vi "WILT Step Drying Clothes 3.vi"(6 "Delay After Cutout (sec)":dbl=5.0 format="%#_13g", 7 "Station Number in":u32, 8 "Error In":errorcluster, 9 "Current Threshold":dbl=1.0 format="%#_13g", 10 "Station Test State Cluster":T1, 11 "Dryer Input":T3 {"Night Cycle Count" format="%04d"; "Day Cycle Count" format="%04d"}) -> (0 "Error Out":errorcluster, 2 "Step 2 Output":T1, 3 "Dryer Output":T3 {"Night Cycle Count" format="%04d"; "Day Cycle Count" format="%04d"})   [LabVIEW 2016]
uses:
  Type Definitions/WILT Dryer.ctl
  Type Definitions/WILT Dryer Details.ctl
  Type Definitions/WILT Agilent Channel Definition.ctl
  Type Definitions/WILT DAQ Data.ctl
  Type Definitions/WILT Station Test State Cluster.ctl
  Type Definitions/WILT Dryer Test State.ctl
  Globals/WILT Globals Main Program.vi
panel:
  # "Day"
  # "Night"
  # "Day"
  # "Night"
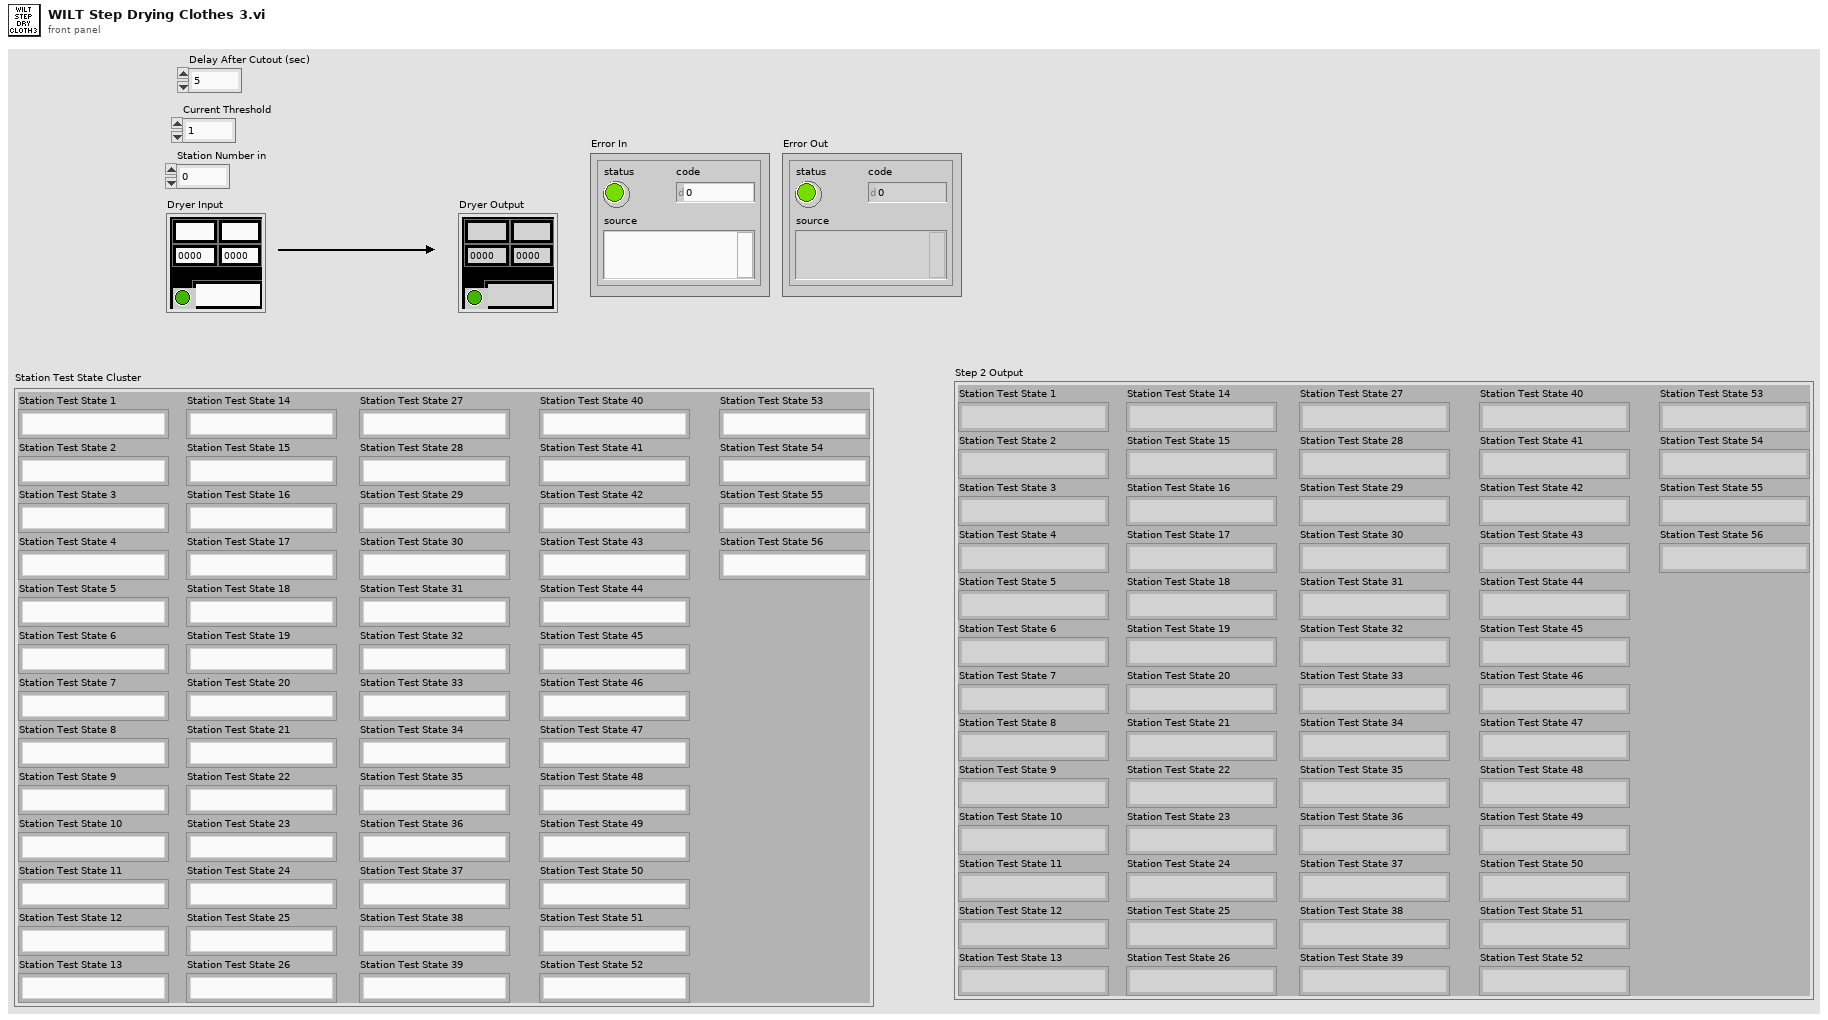
[diagram p1: front panel]
types:
  T1 = typedef "WILT Station Test State Cluster.ctl" = cluster{"Station Test State 1":T2, "Station Test State 2":T2, "Station Test State 3":T2, "Station Test State 4":T2, "Station Test State 5":T2, "Station Test State 6":T2, "Station Test State 7":T2, "Station Test State 8":T2, "Station Test State 9":T2, "Station Test State 10":T2, "Station Test State 11":T2, "Station Test State 12":T2, "Station Test State 13":T2, "Station Test State 14":T2, "Station Test State 15":T2, "Station Test State 16":T2, "Station Test State 17":T2, "Station Test State 18":T2, "Station Test State 19":T2, "Station Test State 20":T2, "Station Test State 21":T2, "Station Test State 22":T2, "Station Test State 23":T2, "Station Test State 24":T2, "Station Test State 25":T2, "Station Test State 26":T2, "Station Test State 27":T2, "Station Test State 28":T2, "Station Test State 29":T2, "Station Test State 30":T2, "Station Test State 31":T2, "Station Test State 32":T2, "Station Test State 33":T2, "Station Test State 34":T2, "Station Test State 35":T2, "Station Test State 36":T2, "Station Test State 37":T2, "Station Test State 38":T2, "Station Test State 39":T2, "Station Test State 40":T2, "Station Test State 41":T2, "Station Test State 42":T2, "Station Test State 43":T2, "Station Test State 44":T2, "Station Test State 45":T2, "Station Test State 46":T2, "Station Test State 47":T2, "Station Test State 48":T2, "Station Test State 49":T2, "Station Test State 50":T2, "Station Test State 51":T2, "Station Test State 52":T2, "Station Test State 53":T2, "Station Test State 54":T2, "Station Test State 55":T2, "Station Test State 56":T2}
  T2 = typedef "WILT Dryer Test State.ctl" = enum16{"No Serial Number", "Waiting for Dryer To Start", "Drying Clothes", "Water Injection 1 (On)", "Water Injection 1 Timer", "Water Injection 1 (Off)", "Pause Dryer", "Sending Start Stop CMD", "Pause Dryer 2", "Sending Start Stop CMD 2", "Drying Clothes 2", "Water Injection 2 (On)", "Water Injection 2 Timer", "Water Injection 2 (Off)", "Drying Clothes 3", "Cooling Down", "Sending Start Stop CMD 3", "Increment Cycle"}
  T3 = typedef "WILT Dryer.ctl" = cluster{"Lab ID":string, "Day Cycle Count":i32, "Station Label":string, "Dryer Details":T4, "Status Color":u32, "Invisible Button":bool, "Night Cycle Count":i32, "Station Index":i32, "Cycle Index":string, "Audit Alert":bool, "Agilent Channel Definition":T5, "DAQ Data":T6}
  T4 = typedef "WILT Dryer Details.ctl" = cluster{"Station":string, "Lab ID":string, "TR Number":string}
  T5 = typedef "WILT Agilent Channel Definition.ctl" = cluster{"Channel":string, "Station":string, "Label":string, "Agilent Station":string, "Data":dbl}
  T6 = typedef "WILT DAQ Data.ctl" = cluster{"L1 Current":dbl, "L2 Current":dbl, "Temperature  Deg F (TC)":dbl, "Volts":dbl, "Volts (208)":dbl, "SW (208)":dbl}
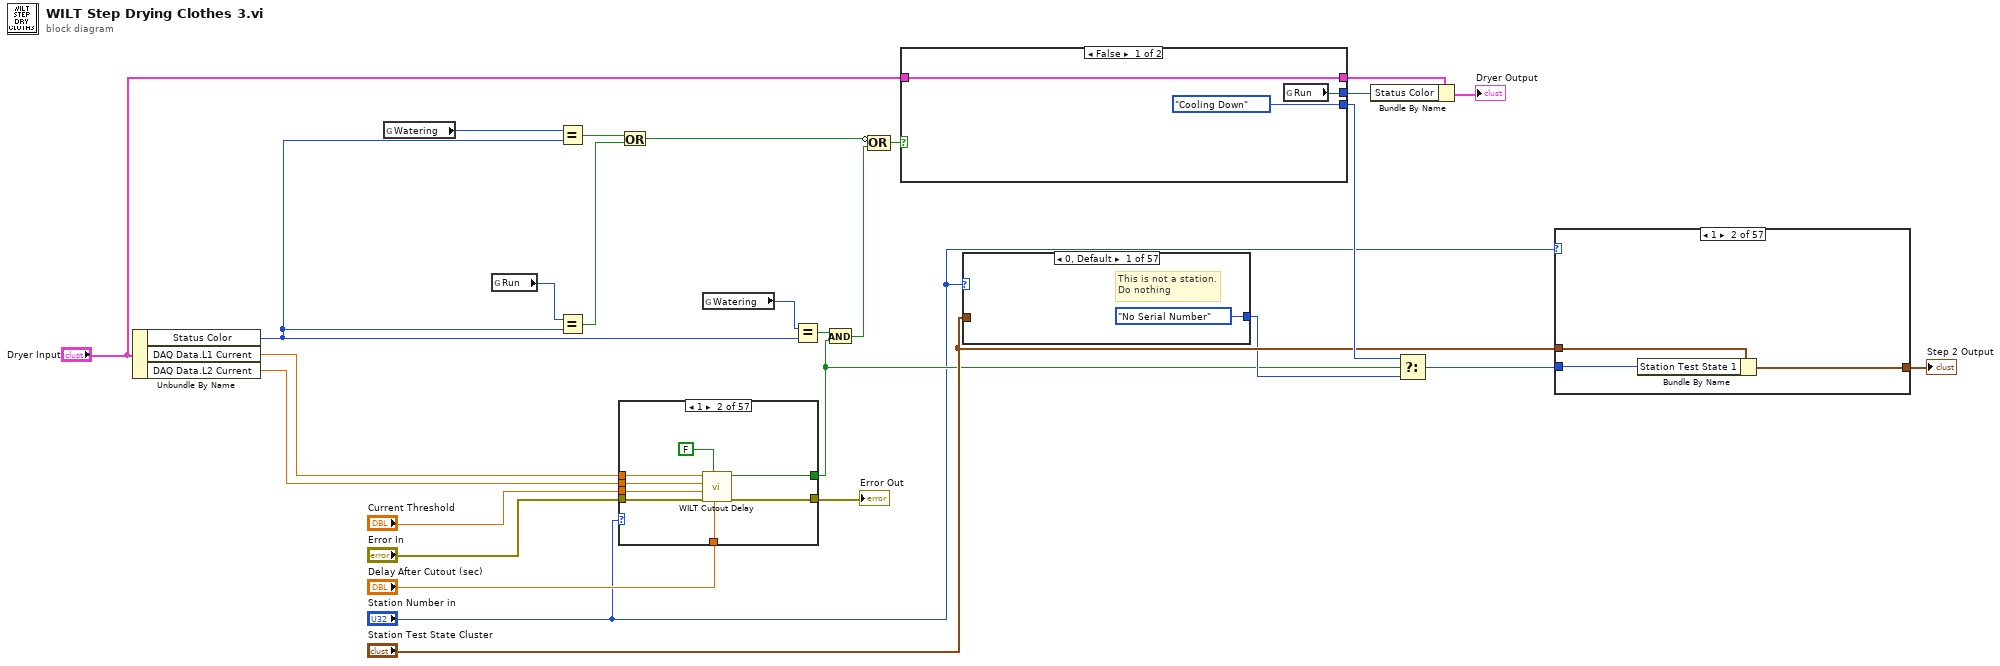
[diagram p0: block diagram]
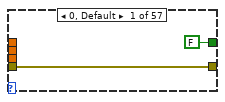
[diagram p2: hidden frame]
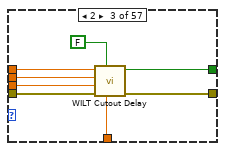
[diagram p3: hidden frame]
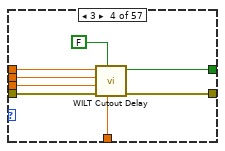
[diagram p4: hidden frame]
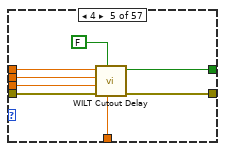
[diagram p5: hidden frame]
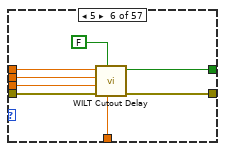
[diagram p6: hidden frame]
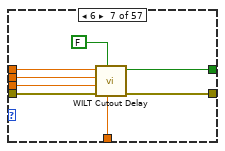
[diagram p7: hidden frame]
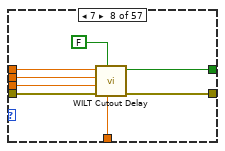
[diagram p8: hidden frame]
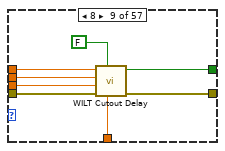
[diagram p9: hidden frame]
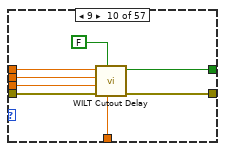
[diagram p10: hidden frame]
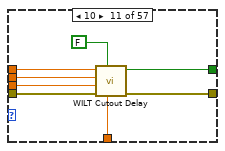
[diagram p11: hidden frame]
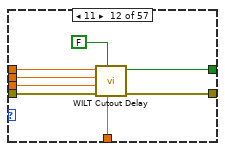
[diagram p12: hidden frame]
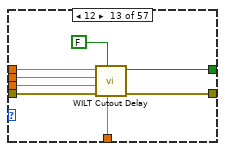
[diagram p13: hidden frame]
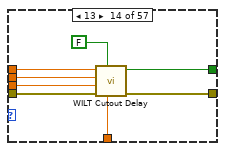
[diagram p14: hidden frame]
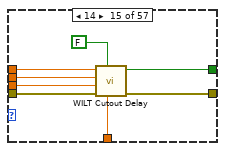
[diagram p15: hidden frame]
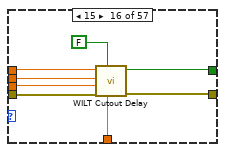
[diagram p16: hidden frame]
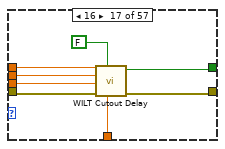
[diagram p17: hidden frame]
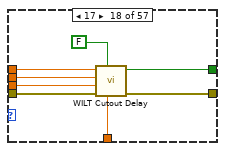
[diagram p18: hidden frame]
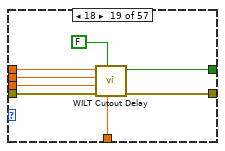
[diagram p19: hidden frame]
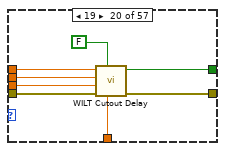
[diagram p20: hidden frame]
diagram:
  n1 = Unbundle By Name("Dryer Input") -> ("Status Color"=w11:u32, "DAQ Data.L1 Current"=w25:dbl, "DAQ Data.L2 Current"=w24:dbl)
  n2 = global read "WILT Globals Main Program.vi" "Watering"() -> (w13:u32)
  n3 = global read "WILT Globals Main Program.vi" "Run"() -> (w12:u32)
  n4 = Equal?(x=w13, y=w11) -> (x = y?=w10:bool)
  n5 = Equal?(x=w12, y=w11) -> (x = y?=w9:bool)
  n6 = case shown="1" "Station Number in" {
    tunnel: "Current Threshold" -> [_ w37 w40 w48 w59 w67 w75 w83 w91 w99 w107 w115 w123 w131 w139 w144 w155 w163 w171 w179 w187 w195 w203 w211 w219 w227 w235 w243 w251 w259 w267 w275 w283 w291 w299 w307 w315 w323 w331 w339 w347 w355 w363 w371 w379 w387 w395 w403 w411 w419 w427 w435 w443 w451 w459 w467 w475]
    tunnel: w25 -> [_ w36 w42 w50 w61 w69 w77 w85 w93 w101 w109 w117 w125 w133 w141 w146 w157 w165 w173 w181 w189 w197 w205 w213 w221 w229 w237 w245 w253 w261 w269 w277 w285 w293 w301 w309 w317 w325 w333 w341 w349 w357 w365 w373 w381 w389 w397 w405 w413 w421 w429 w437 w445 w453 w461 w469 w477]
    tunnel: w24 -> [_ w35 w41 w49 w60 w68 w76 w84 w92 w100 w108 w116 w124 w132 w140 w145 w156 w164 w172 w180 w188 w196 w204 w212 w220 w228 w236 w244 w252 w260 w268 w276 w284 w292 w300 w308 w316 w324 w332 w340 w348 w356 w364 w372 w380 w388 w396 w404 w412 w420 w428 w436 w444 w452 w460 w468 w476]
    tunnel: [FALSE ("Delayed Trigger") w34 w39 w51 w55 w64 w72 w79 w88 w96 w104 w111 w121 w129 w137 w147 w152 w160 w168 w177 w184 w191 w200 w207 w216 w224 w231 w240 w248 w256 w264 w271 w279 w287 w295 w303 w312 w319 w327 w336 w343 w351 w359 w367 w376 w384 w391 w400 w407 w416 w424 w432 w440 w448 w456 w464 w471] -> w16
    tunnel: "Error In" -> [w29 w33 w45 w53 w58 w66 w74 w82 w90 w98 w106 w114 w122 w130 w138 w149 w154 w162 w170 w178 w186 w194 w202 w210 w218 w226 w234 w242 w250 w258 w266 w274 w282 w290 w298 w306 w314 w322 w330 w338 w346 w354 w362 w370 w378 w386 w394 w402 w410 w418 w426 w434 w442 w450 w458 w466 w474]
    tunnel: [w29 w32 w44 w52 w56 w65 w71 w80 w89 w97 w103 w112 w120 w128 w136 w148 w153 w161 w169 w176 w185 w192 w199 w208 w217 w223 w232 w241 w249 w257 w265 w272 w280 w288 w296 w304 w313 w320 w328 w337 w344 w352 w360 w368 w377 w385 w392 w401 w408 w417 w425 w433 w441 w449 w457 w465 w472] -> w3
    tunnel: "Delay After Cutout (sec)" -> [_ w31 w43 w47 w57 w63 w73 w81 w87 w95 w105 w113 w119 w127 w135 w143 w151 w159 w167 w175 w183 w193 w201 w209 w215 w225 w233 w239 w247 w255 w263 w273 w281 w289 w297 w305 w311 w321 w329 w335 w345 w353 w361 w369 w375 w383 w393 w399 w409 w415 w423 w431 w439 w447 w455 w463 w473]
    frame 0, Default {
    }
    frame 1 {
      n7 = call "WILT Cutout Delay.vi"("Delay After Cutout (sec)"=w31, "Cut-In?"=FALSE, "Error In"=w33, "Current Threshold"=w37, "L2 Current"=w35, "L1 Current"=w36) -> ("Error Out"=w32:errorcluster, "Delayed Trigger"=w34:bool)  [unwired: 2 in, 2 out]
    }
    frame 2 {
      n8 = call "WILT Cutout Delay.vi"("Delay After Cutout (sec)"=w43, "Cut-In?"=FALSE, "Error In"=w45, "Current Threshold"=w40, "L2 Current"=w41, "L1 Current"=w42) -> ("Error Out"=w44:errorcluster, "Delayed Trigger"=w39:bool)  [unwired: 2 in, 2 out]
    }
    frame 3 {
      n9 = call "WILT Cutout Delay.vi"("Delay After Cutout (sec)"=w47, "Cut-In?"=FALSE, "Error In"=w53, "Current Threshold"=w48, "L2 Current"=w49, "L1 Current"=w50) -> ("Error Out"=w52:errorcluster, "Delayed Trigger"=w51:bool)  [unwired: 2 in, 2 out]
    }
    frame 4 {
      n10 = call "WILT Cutout Delay.vi"("Delay After Cutout (sec)"=w57, "Cut-In?"=FALSE, "Error In"=w58, "Current Threshold"=w59, "L2 Current"=w60, "L1 Current"=w61) -> ("Error Out"=w56:errorcluster, "Delayed Trigger"=w55:bool)  [unwired: 2 in, 2 out]
    }
    frame 5 {
      n11 = call "WILT Cutout Delay.vi"("Delay After Cutout (sec)"=w63, "Cut-In?"=FALSE, "Error In"=w66, "Current Threshold"=w67, "L2 Current"=w68, "L1 Current"=w69) -> ("Error Out"=w65:errorcluster, "Delayed Trigger"=w64:bool)  [unwired: 2 in, 2 out]
    }
    frame 6 {
      n12 = call "WILT Cutout Delay.vi"("Delay After Cutout (sec)"=w73, "Cut-In?"=FALSE, "Error In"=w74, "Current Threshold"=w75, "L2 Current"=w76, "L1 Current"=w77) -> ("Error Out"=w71:errorcluster, "Delayed Trigger"=w72:bool)  [unwired: 2 in, 2 out]
    }
    frame 7 {
      n13 = call "WILT Cutout Delay.vi"("Delay After Cutout (sec)"=w81, "Cut-In?"=FALSE, "Error In"=w82, "Current Threshold"=w83, "L2 Current"=w84, "L1 Current"=w85) -> ("Error Out"=w80:errorcluster, "Delayed Trigger"=w79:bool)  [unwired: 2 in, 2 out]
    }
    frame 8 {
      n14 = call "WILT Cutout Delay.vi"("Delay After Cutout (sec)"=w87, "Cut-In?"=FALSE, "Error In"=w90, "Current Threshold"=w91, "L2 Current"=w92, "L1 Current"=w93) -> ("Error Out"=w89:errorcluster, "Delayed Trigger"=w88:bool)  [unwired: 2 in, 2 out]
    }
    frame 9 {
      n15 = call "WILT Cutout Delay.vi"("Delay After Cutout (sec)"=w95, "Cut-In?"=FALSE, "Error In"=w98, "Current Threshold"=w99, "L2 Current"=w100, "L1 Current"=w101) -> ("Error Out"=w97:errorcluster, "Delayed Trigger"=w96:bool)  [unwired: 2 in, 2 out]
    }
    frame 10 {
      n16 = call "WILT Cutout Delay.vi"("Delay After Cutout (sec)"=w105, "Cut-In?"=FALSE, "Error In"=w106, "Current Threshold"=w107, "L2 Current"=w108, "L1 Current"=w109) -> ("Error Out"=w103:errorcluster, "Delayed Trigger"=w104:bool)  [unwired: 2 in, 2 out]
    }
    frame 11 {
      n17 = call "WILT Cutout Delay.vi"("Delay After Cutout (sec)"=w113, "Cut-In?"=FALSE, "Error In"=w114, "Current Threshold"=w115, "L2 Current"=w116, "L1 Current"=w117) -> ("Error Out"=w112:errorcluster, "Delayed Trigger"=w111:bool)  [unwired: 2 in, 2 out]
    }
    frame 12 {
      n18 = call "WILT Cutout Delay.vi"("Delay After Cutout (sec)"=w119, "Cut-In?"=FALSE, "Error In"=w122, "Current Threshold"=w123, "L2 Current"=w124, "L1 Current"=w125) -> ("Error Out"=w120:errorcluster, "Delayed Trigger"=w121:bool)  [unwired: 2 in, 2 out]
    }
    frame 13 {
      n19 = call "WILT Cutout Delay.vi"("Delay After Cutout (sec)"=w127, "Cut-In?"=FALSE, "Error In"=w130, "Current Threshold"=w131, "L2 Current"=w132, "L1 Current"=w133) -> ("Error Out"=w128:errorcluster, "Delayed Trigger"=w129:bool)  [unwired: 2 in, 2 out]
    }
    frame 14 {
      n20 = call "WILT Cutout Delay.vi"("Delay After Cutout (sec)"=w135, "Cut-In?"=FALSE, "Error In"=w138, "Current Threshold"=w139, "L2 Current"=w140, "L1 Current"=w141) -> ("Error Out"=w136:errorcluster, "Delayed Trigger"=w137:bool)  [unwired: 2 in, 2 out]
    }
    frame 15 {
      n21 = call "WILT Cutout Delay.vi"("Delay After Cutout (sec)"=w143, "Cut-In?"=FALSE, "Error In"=w149, "Current Threshold"=w144, "L2 Current"=w145, "L1 Current"=w146) -> ("Error Out"=w148:errorcluster, "Delayed Trigger"=w147:bool)  [unwired: 2 in, 2 out]
    }
    frame 16 {
      n22 = call "WILT Cutout Delay.vi"("Delay After Cutout (sec)"=w151, "Cut-In?"=FALSE, "Error In"=w154, "Current Threshold"=w155, "L2 Current"=w156, "L1 Current"=w157) -> ("Error Out"=w153:errorcluster, "Delayed Trigger"=w152:bool)  [unwired: 2 in, 2 out]
    }
    frame 17 {
      n23 = call "WILT Cutout Delay.vi"("Delay After Cutout (sec)"=w159, "Cut-In?"=FALSE, "Error In"=w162, "Current Threshold"=w163, "L2 Current"=w164, "L1 Current"=w165) -> ("Error Out"=w161:errorcluster, "Delayed Trigger"=w160:bool)  [unwired: 2 in, 2 out]
    }
    frame 18 {
      n24 = call "WILT Cutout Delay.vi"("Delay After Cutout (sec)"=w167, "Cut-In?"=FALSE, "Error In"=w170, "Current Threshold"=w171, "L2 Current"=w172, "L1 Current"=w173) -> ("Error Out"=w169:errorcluster, "Delayed Trigger"=w168:bool)  [unwired: 2 in, 2 out]
    }
    frame 19 {
      n25 = call "WILT Cutout Delay.vi"("Delay After Cutout (sec)"=w175, "Cut-In?"=FALSE, "Error In"=w178, "Current Threshold"=w179, "L2 Current"=w180, "L1 Current"=w181) -> ("Error Out"=w176:errorcluster, "Delayed Trigger"=w177:bool)  [unwired: 2 in, 2 out]
    }
    frame 20 {
      n26 = call "WILT Cutout Delay.vi"("Delay After Cutout (sec)"=w183, "Cut-In?"=FALSE, "Error In"=w186, "Current Threshold"=w187, "L2 Current"=w188, "L1 Current"=w189) -> ("Error Out"=w185:errorcluster, "Delayed Trigger"=w184:bool)  [unwired: 2 in, 2 out]
    }
    frame 21 {
      n27 = call "WILT Cutout Delay.vi"("Delay After Cutout (sec)"=w193, "Cut-In?"=FALSE, "Error In"=w194, "Current Threshold"=w195, "L2 Current"=w196, "L1 Current"=w197) -> ("Error Out"=w192:errorcluster, "Delayed Trigger"=w191:bool)  [unwired: 2 in, 2 out]
    }
    frame 22 {
      n28 = call "WILT Cutout Delay.vi"("Delay After Cutout (sec)"=w201, "Cut-In?"=FALSE, "Error In"=w202, "Current Threshold"=w203, "L2 Current"=w204, "L1 Current"=w205) -> ("Error Out"=w199:errorcluster, "Delayed Trigger"=w200:bool)  [unwired: 2 in, 2 out]
    }
    frame 23 {
      n29 = call "WILT Cutout Delay.vi"("Delay After Cutout (sec)"=w209, "Cut-In?"=FALSE, "Error In"=w210, "Current Threshold"=w211, "L2 Current"=w212, "L1 Current"=w213) -> ("Error Out"=w208:errorcluster, "Delayed Trigger"=w207:bool)  [unwired: 2 in, 2 out]
    }
    frame 24 {
      n30 = call "WILT Cutout Delay.vi"("Delay After Cutout (sec)"=w215, "Cut-In?"=FALSE, "Error In"=w218, "Current Threshold"=w219, "L2 Current"=w220, "L1 Current"=w221) -> ("Error Out"=w217:errorcluster, "Delayed Trigger"=w216:bool)  [unwired: 2 in, 2 out]
    }
    frame 25 {
      n31 = call "WILT Cutout Delay.vi"("Delay After Cutout (sec)"=w225, "Cut-In?"=FALSE, "Error In"=w226, "Current Threshold"=w227, "L2 Current"=w228, "L1 Current"=w229) -> ("Error Out"=w223:errorcluster, "Delayed Trigger"=w224:bool)  [unwired: 2 in, 2 out]
    }
    frame 26 {
      n32 = call "WILT Cutout Delay.vi"("Delay After Cutout (sec)"=w233, "Cut-In?"=FALSE, "Error In"=w234, "Current Threshold"=w235, "L2 Current"=w236, "L1 Current"=w237) -> ("Error Out"=w232:errorcluster, "Delayed Trigger"=w231:bool)  [unwired: 2 in, 2 out]
    }
    frame 27 {
      n33 = call "WILT Cutout Delay.vi"("Delay After Cutout (sec)"=w239, "Cut-In?"=FALSE, "Error In"=w242, "Current Threshold"=w243, "L2 Current"=w244, "L1 Current"=w245) -> ("Error Out"=w241:errorcluster, "Delayed Trigger"=w240:bool)  [unwired: 2 in, 2 out]
    }
    frame 28 {
      n34 = call "WILT Cutout Delay.vi"("Delay After Cutout (sec)"=w247, "Cut-In?"=FALSE, "Error In"=w250, "Current Threshold"=w251, "L2 Current"=w252, "L1 Current"=w253) -> ("Error Out"=w249:errorcluster, "Delayed Trigger"=w248:bool)  [unwired: 2 in, 2 out]
    }
    frame 29 {
      n35 = call "WILT Cutout Delay.vi"("Delay After Cutout (sec)"=w255, "Cut-In?"=FALSE, "Error In"=w258, "Current Threshold"=w259, "L2 Current"=w260, "L1 Current"=w261) -> ("Error Out"=w257:errorcluster, "Delayed Trigger"=w256:bool)  [unwired: 2 in, 2 out]
    }
    frame 30 {
      n36 = call "WILT Cutout Delay.vi"("Delay After Cutout (sec)"=w263, "Cut-In?"=FALSE, "Error In"=w266, "Current Threshold"=w267, "L2 Current"=w268, "L1 Current"=w269) -> ("Error Out"=w265:errorcluster, "Delayed Trigger"=w264:bool)  [unwired: 2 in, 2 out]
    }
    frame 31 {
      n37 = call "WILT Cutout Delay.vi"("Delay After Cutout (sec)"=w273, "Cut-In?"=FALSE, "Error In"=w274, "Current Threshold"=w275, "L2 Current"=w276, "L1 Current"=w277) -> ("Error Out"=w272:errorcluster, "Delayed Trigger"=w271:bool)  [unwired: 2 in, 2 out]
    }
    frame 32 {
      n38 = call "WILT Cutout Delay.vi"("Delay After Cutout (sec)"=w281, "Cut-In?"=FALSE, "Error In"=w282, "Current Threshold"=w283, "L2 Current"=w284, "L1 Current"=w285) -> ("Error Out"=w280:errorcluster, "Delayed Trigger"=w279:bool)  [unwired: 2 in, 2 out]
    }
    frame 33 {
      n39 = call "WILT Cutout Delay.vi"("Delay After Cutout (sec)"=w289, "Cut-In?"=FALSE, "Error In"=w290, "Current Threshold"=w291, "L2 Current"=w292, "L1 Current"=w293) -> ("Error Out"=w288:errorcluster, "Delayed Trigger"=w287:bool)  [unwired: 2 in, 2 out]
    }
    frame 34 {
      n40 = call "WILT Cutout Delay.vi"("Delay After Cutout (sec)"=w297, "Cut-In?"=FALSE, "Error In"=w298, "Current Threshold"=w299, "L2 Current"=w300, "L1 Current"=w301) -> ("Error Out"=w296:errorcluster, "Delayed Trigger"=w295:bool)  [unwired: 2 in, 2 out]
    }
    frame 35 {
      n41 = call "WILT Cutout Delay.vi"("Delay After Cutout (sec)"=w305, "Cut-In?"=FALSE, "Error In"=w306, "Current Threshold"=w307, "L2 Current"=w308, "L1 Current"=w309) -> ("Error Out"=w304:errorcluster, "Delayed Trigger"=w303:bool)  [unwired: 2 in, 2 out]
    }
    frame 36 {
      n42 = call "WILT Cutout Delay.vi"("Delay After Cutout (sec)"=w311, "Cut-In?"=FALSE, "Error In"=w314, "Current Threshold"=w315, "L2 Current"=w316, "L1 Current"=w317) -> ("Error Out"=w313:errorcluster, "Delayed Trigger"=w312:bool)  [unwired: 2 in, 2 out]
    }
    frame 37 {
      n43 = call "WILT Cutout Delay.vi"("Delay After Cutout (sec)"=w321, "Cut-In?"=FALSE, "Error In"=w322, "Current Threshold"=w323, "L2 Current"=w324, "L1 Current"=w325) -> ("Error Out"=w320:errorcluster, "Delayed Trigger"=w319:bool)  [unwired: 2 in, 2 out]
    }
    frame 38 {
      n44 = call "WILT Cutout Delay.vi"("Delay After Cutout (sec)"=w329, "Cut-In?"=FALSE, "Error In"=w330, "Current Threshold"=w331, "L2 Current"=w332, "L1 Current"=w333) -> ("Error Out"=w328:errorcluster, "Delayed Trigger"=w327:bool)  [unwired: 2 in, 2 out]
    }
    frame 39 {
      n45 = call "WILT Cutout Delay.vi"("Delay After Cutout (sec)"=w335, "Cut-In?"=FALSE, "Error In"=w338, "Current Threshold"=w339, "L2 Current"=w340, "L1 Current"=w341) -> ("Error Out"=w337:errorcluster, "Delayed Trigger"=w336:bool)  [unwired: 2 in, 2 out]
    }
    frame 40 {
      n46 = call "WILT Cutout Delay.vi"("Delay After Cutout (sec)"=w345, "Cut-In?"=FALSE, "Error In"=w346, "Current Threshold"=w347, "L2 Current"=w348, "L1 Current"=w349) -> ("Error Out"=w344:errorcluster, "Delayed Trigger"=w343:bool)  [unwired: 2 in, 2 out]
    }
    frame 41 {
      n47 = call "WILT Cutout Delay.vi"("Delay After Cutout (sec)"=w353, "Cut-In?"=FALSE, "Error In"=w354, "Current Threshold"=w355, "L2 Current"=w356, "L1 Current"=w357) -> ("Error Out"=w352:errorcluster, "Delayed Trigger"=w351:bool)  [unwired: 2 in, 2 out]
    }
    frame 42 {
      n48 = call "WILT Cutout Delay.vi"("Delay After Cutout (sec)"=w361, "Cut-In?"=FALSE, "Error In"=w362, "Current Threshold"=w363, "L2 Current"=w364, "L1 Current"=w365) -> ("Error Out"=w360:errorcluster, "Delayed Trigger"=w359:bool)  [unwired: 2 in, 2 out]
    }
    frame 43 {
      n49 = call "WILT Cutout Delay.vi"("Delay After Cutout (sec)"=w369, "Cut-In?"=FALSE, "Error In"=w370, "Current Threshold"=w371, "L2 Current"=w372, "L1 Current"=w373) -> ("Error Out"=w368:errorcluster, "Delayed Trigger"=w367:bool)  [unwired: 2 in, 2 out]
    }
    frame 44 {
      n50 = call "WILT Cutout Delay.vi"("Delay After Cutout (sec)"=w375, "Cut-In?"=FALSE, "Error In"=w378, "Current Threshold"=w379, "L2 Current"=w380, "L1 Current"=w381) -> ("Error Out"=w377:errorcluster, "Delayed Trigger"=w376:bool)  [unwired: 2 in, 2 out]
    }
    frame 45 {
      n51 = call "WILT Cutout Delay.vi"("Delay After Cutout (sec)"=w383, "Cut-In?"=FALSE, "Error In"=w386, "Current Threshold"=w387, "L2 Current"=w388, "L1 Current"=w389) -> ("Error Out"=w385:errorcluster, "Delayed Trigger"=w384:bool)  [unwired: 2 in, 2 out]
    }
    frame 46 {
      n52 = call "WILT Cutout Delay.vi"("Delay After Cutout (sec)"=w393, "Cut-In?"=FALSE, "Error In"=w394, "Current Threshold"=w395, "L2 Current"=w396, "L1 Current"=w397) -> ("Error Out"=w392:errorcluster, "Delayed Trigger"=w391:bool)  [unwired: 2 in, 2 out]
    }
    frame 47 {
      n53 = call "WILT Cutout Delay.vi"("Delay After Cutout (sec)"=w399, "Cut-In?"=FALSE, "Error In"=w402, "Current Threshold"=w403, "L2 Current"=w404, "L1 Current"=w405) -> ("Error Out"=w401:errorcluster, "Delayed Trigger"=w400:bool)  [unwired: 2 in, 2 out]
    }
    frame 48 {
      n54 = call "WILT Cutout Delay.vi"("Delay After Cutout (sec)"=w409, "Cut-In?"=FALSE, "Error In"=w410, "Current Threshold"=w411, "L2 Current"=w412, "L1 Current"=w413) -> ("Error Out"=w408:errorcluster, "Delayed Trigger"=w407:bool)  [unwired: 2 in, 2 out]
    }
    frame 49 {
      n55 = call "WILT Cutout Delay.vi"("Delay After Cutout (sec)"=w415, "Cut-In?"=FALSE, "Error In"=w418, "Current Threshold"=w419, "L2 Current"=w420, "L1 Current"=w421) -> ("Error Out"=w417:errorcluster, "Delayed Trigger"=w416:bool)  [unwired: 2 in, 2 out]
    }
    frame 50 {
      n56 = call "WILT Cutout Delay.vi"("Delay After Cutout (sec)"=w423, "Cut-In?"=FALSE, "Error In"=w426, "Current Threshold"=w427, "L2 Current"=w428, "L1 Current"=w429) -> ("Error Out"=w425:errorcluster, "Delayed Trigger"=w424:bool)  [unwired: 2 in, 2 out]
    }
    frame 51 {
      n57 = call "WILT Cutout Delay.vi"("Delay After Cutout (sec)"=w431, "Cut-In?"=FALSE, "Error In"=w434, "Current Threshold"=w435, "L2 Current"=w436, "L1 Current"=w437) -> ("Error Out"=w433:errorcluster, "Delayed Trigger"=w432:bool)  [unwired: 2 in, 2 out]
    }
    frame 52 {
      n58 = call "WILT Cutout Delay.vi"("Delay After Cutout (sec)"=w439, "Cut-In?"=FALSE, "Error In"=w442, "Current Threshold"=w443, "L2 Current"=w444, "L1 Current"=w445) -> ("Error Out"=w441:errorcluster, "Delayed Trigger"=w440:bool)  [unwired: 2 in, 2 out]
    }
    frame 53 {
      n59 = call "WILT Cutout Delay.vi"("Delay After Cutout (sec)"=w447, "Cut-In?"=FALSE, "Error In"=w450, "Current Threshold"=w451, "L2 Current"=w452, "L1 Current"=w453) -> ("Error Out"=w449:errorcluster, "Delayed Trigger"=w448:bool)  [unwired: 2 in, 2 out]
    }
    frame 54 {
      n60 = call "WILT Cutout Delay.vi"("Delay After Cutout (sec)"=w455, "Cut-In?"=FALSE, "Error In"=w458, "Current Threshold"=w459, "L2 Current"=w460, "L1 Current"=w461) -> ("Error Out"=w457:errorcluster, "Delayed Trigger"=w456:bool)  [unwired: 2 in, 2 out]
    }
    frame 55 {
      n61 = call "WILT Cutout Delay.vi"("Delay After Cutout (sec)"=w463, "Cut-In?"=FALSE, "Error In"=w466, "Current Threshold"=w467, "L2 Current"=w468, "L1 Current"=w469) -> ("Error Out"=w465:errorcluster, "Delayed Trigger"=w464:bool)  [unwired: 2 in, 2 out]
    }
    frame 56 {
      n62 = call "WILT Cutout Delay.vi"("Delay After Cutout (sec)"=w473, "Cut-In?"=FALSE, "Error In"=w474, "Current Threshold"=w475, "L2 Current"=w476, "L1 Current"=w477) -> ("Error Out"=w472:errorcluster, "Delayed Trigger"=w471:bool)  [unwired: 2 in, 2 out]
    }
  }
  "Error Out" <- w3
  n63 = Or(x=w10, y=w9) -> (x .or. y?=w7:bool)
  n64 = global read "WILT Globals Main Program.vi" "Watering"() -> (w18:u32)
  n65 = Equal?(x=w18, y=w11) -> (x = y?=w17:bool)
  n66 = And(x=w17, y=w16) -> (x .and. y?=w8:bool)
  n67 = Compound Arithmetic op=OR(invert w7, w8) -> (w6:bool)
  n68 = case shown="False" w6 {
    tunnel: [WILT_Dryer_Test_State."Cooling Down" ("Station Test State Input 2") WILT_Dryer_Test_State."No Serial Number" ("Station Test State Input 2")] -> w23
    tunnel: "Dryer Input" -> [w479 w482]
    tunnel: [w479 w482] -> w15
    tunnel: [w478 w481] -> w14
    frame False {
      n69 = global read "WILT Globals Main Program.vi" "Run"() -> (w478:u32)
    }
    frame True {
      n70 = global read "WILT Globals Main Program.vi" "EOC"() -> (w481:u32)
    }
  }
  n71 = case shown="0, Default" "Station Number in" {
    tunnel: "Station Test State Cluster" -> [_ w486 w488 w490 w492 w494 w496 w498 w500 w502 w504 w506 w508 w510 w512 w514 w516 w518 w520 w522 w524 w526 w528 w530 w532 w534 w536 w538 w540 w542 w544 w546 w548 w550 w552 w554 w556 w558 w560 w562 w564 w566 w568 w570 w572 w574 w576 w578 w580 w582 w584 w586 w588 w590 w592 w594 w596]
    tunnel: [WILT_Dryer_Test_State."No Serial Number" ("Station Test State 56") w485 w487 w489 w491 w493 w495 w497 w499 w501 w503 w505 w507 w509 w511 w513 w515 w517 w519 w521 w523 w525 w527 w529 w531 w533 w535 w537 w539 w541 w543 w545 w547 w549 w551 w553 w555 w557 w559 w561 w563 w565 w567 w569 w571 w573 w575 w577 w579 w581 w583 w585 w587 w589 w591 w593 w595] -> w20
    frame 0, Default {
      # "This is not a station.\nDo nothing"
    }
    frame 1 {
      n72 = Unbundle By Name(w486) -> ("Station Test State 1"=w485:T2)
    }
    frame 2 {
      n73 = Unbundle By Name(w488) -> ("Station Test State 2"=w487:T2)
    }
    frame 3 {
      n74 = Unbundle By Name(w490) -> ("Station Test State 3"=w489:T2)
    }
    frame 4 {
      n75 = Unbundle By Name(w492) -> ("Station Test State 4"=w491:T2)
    }
    frame 5 {
      n76 = Unbundle By Name(w494) -> ("Station Test State 5"=w493:T2)
    }
    frame 6 {
      n77 = Unbundle By Name(w496) -> ("Station Test State 6"=w495:T2)
    }
    frame 7 {
      n78 = Unbundle By Name(w498) -> ("Station Test State 7"=w497:T2)
    }
    frame 8 {
      n79 = Unbundle By Name(w500) -> ("Station Test State 8"=w499:T2)
    }
    frame 9 {
      n80 = Unbundle By Name(w502) -> ("Station Test State 9"=w501:T2)
    }
    frame 10 {
      n81 = Unbundle By Name(w504) -> ("Station Test State 10"=w503:T2)
    }
    frame 11 {
      n82 = Unbundle By Name(w506) -> ("Station Test State 11"=w505:T2)
    }
    frame 12 {
      n83 = Unbundle By Name(w508) -> ("Station Test State 12"=w507:T2)
    }
    frame 13 {
      n84 = Unbundle By Name(w510) -> ("Station Test State 13"=w509:T2)
    }
    frame 14 {
      n85 = Unbundle By Name(w512) -> ("Station Test State 14"=w511:T2)
    }
    frame 15 {
      n86 = Unbundle By Name(w514) -> ("Station Test State 15"=w513:T2)
    }
    frame 16 {
      n87 = Unbundle By Name(w516) -> ("Station Test State 16"=w515:T2)
    }
    frame 17 {
      n88 = Unbundle By Name(w518) -> ("Station Test State 17"=w517:T2)
    }
    frame 18 {
      n89 = Unbundle By Name(w520) -> ("Station Test State 18"=w519:T2)
    }
    frame 19 {
      n90 = Unbundle By Name(w522) -> ("Station Test State 19"=w521:T2)
    }
    frame 20 {
      n91 = Unbundle By Name(w524) -> ("Station Test State 20"=w523:T2)
    }
    frame 21 {
      n92 = Unbundle By Name(w526) -> ("Station Test State 21"=w525:T2)
    }
    frame 22 {
      n93 = Unbundle By Name(w528) -> ("Station Test State 22"=w527:T2)
    }
    frame 23 {
      n94 = Unbundle By Name(w530) -> ("Station Test State 23"=w529:T2)
    }
    frame 24 {
      n95 = Unbundle By Name(w532) -> ("Station Test State 24"=w531:T2)
    }
    frame 25 {
      n96 = Unbundle By Name(w534) -> ("Station Test State 25"=w533:T2)
    }
    frame 26 {
      n97 = Unbundle By Name(w536) -> ("Station Test State 26"=w535:T2)
    }
    frame 27 {
      n98 = Unbundle By Name(w538) -> ("Station Test State 27"=w537:T2)
    }
    frame 28 {
      n99 = Unbundle By Name(w540) -> ("Station Test State 28"=w539:T2)
    }
    frame 29 {
      n100 = Unbundle By Name(w542) -> ("Station Test State 29"=w541:T2)
    }
    frame 30 {
      n101 = Unbundle By Name(w544) -> ("Station Test State 30"=w543:T2)
    }
    frame 31 {
      n102 = Unbundle By Name(w546) -> ("Station Test State 31"=w545:T2)
    }
    frame 32 {
      n103 = Unbundle By Name(w548) -> ("Station Test State 32"=w547:T2)
    }
    frame 33 {
      n104 = Unbundle By Name(w550) -> ("Station Test State 33"=w549:T2)
    }
    frame 34 {
      n105 = Unbundle By Name(w552) -> ("Station Test State 34"=w551:T2)
    }
    frame 35 {
      n106 = Unbundle By Name(w554) -> ("Station Test State 35"=w553:T2)
    }
    frame 36 {
      n107 = Unbundle By Name(w556) -> ("Station Test State 36"=w555:T2)
    }
    frame 37 {
      n108 = Unbundle By Name(w558) -> ("Station Test State 37"=w557:T2)
    }
    frame 38 {
      n109 = Unbundle By Name(w560) -> ("Station Test State 38"=w559:T2)
    }
    frame 39 {
      n110 = Unbundle By Name(w562) -> ("Station Test State 39"=w561:T2)
    }
    frame 40 {
      n111 = Unbundle By Name(w564) -> ("Station Test State 40"=w563:T2)
    }
    frame 41 {
      n112 = Unbundle By Name(w566) -> ("Station Test State 41"=w565:T2)
    }
    frame 42 {
      n113 = Unbundle By Name(w568) -> ("Station Test State 42"=w567:T2)
    }
    frame 43 {
      n114 = Unbundle By Name(w570) -> ("Station Test State 43"=w569:T2)
    }
    frame 44 {
      n115 = Unbundle By Name(w572) -> ("Station Test State 44"=w571:T2)
    }
    frame 45 {
      n116 = Unbundle By Name(w574) -> ("Station Test State 45"=w573:T2)
    }
    frame 46 {
      n117 = Unbundle By Name(w576) -> ("Station Test State 46"=w575:T2)
    }
    frame 47 {
      n118 = Unbundle By Name(w578) -> ("Station Test State 47"=w577:T2)
    }
    frame 48 {
      n119 = Unbundle By Name(w580) -> ("Station Test State 48"=w579:T2)
    }
    frame 49 {
      n120 = Unbundle By Name(w582) -> ("Station Test State 49"=w581:T2)
    }
    frame 50 {
      n121 = Unbundle By Name(w584) -> ("Station Test State 50"=w583:T2)
    }
    frame 51 {
      n122 = Unbundle By Name(w586) -> ("Station Test State 51"=w585:T2)
    }
    frame 52 {
      n123 = Unbundle By Name(w588) -> ("Station Test State 52"=w587:T2)
    }
    frame 53 {
      n124 = Unbundle By Name(w590) -> ("Station Test State 53"=w589:T2)
    }
    frame 54 {
      n125 = Unbundle By Name(w592) -> ("Station Test State 54"=w591:T2)
    }
    frame 55 {
      n126 = Unbundle By Name(w594) -> ("Station Test State 55"=w593:T2)
    }
    frame 56 {
      n127 = Unbundle By Name(w596) -> ("Station Test State 56"=w595:T2)
    }
  }
  n128 = Bundle By Name(cluster=w15, "Status Color"=w14) -> (→"Dryer Output":T3)
  n129 = Select(t=w23, s=w16, f=w20) -> (s? t:f=w22:T2)
  n130 = case shown="1" "Station Number in" {
    tunnel: "Station Test State Cluster" -> [w597 w600 w603 w606 w609 w612 w615 w618 w621 w624 w627 w630 w633 w636 w639 w642 w645 w648 w651 w654 w657 w660 w663 w666 w669 w672 w675 w678 w681 w684 w687 w690 w693 w696 w699 w702 w705 w708 w711 w714 w717 w720 w723 w726 w729 w732 w735 w738 w741 w744 w747 w750 w753 w756 w759 w762 w765]
    tunnel: w22 -> [_ w599 w601 w604 w607 w610 w613 w616 w619 w622 w625 w628 w631 w634 w637 w640 w643 w646 w649 w652 w655 w658 w661 w664 w667 w670 w673 w676 w679 w682 w685 w688 w691 w694 w697 w700 w703 w706 w709 w712 w715 w718 w721 w724 w727 w730 w733 w736 w739 w742 w745 w748 w751 w754 w757 w760 w763]
    tunnel: [w597 w598 w602 w605 w608 w611 w614 w617 w620 w623 w626 w629 w632 w635 w638 w641 w644 w647 w650 w653 w656 w659 w662 w665 w668 w671 w674 w677 w680 w683 w686 w689 w692 w695 w698 w701 w704 w707 w710 w713 w716 w719 w722 w725 w728 w731 w734 w737 w740 w743 w746 w749 w752 w755 w758 w761 w764] -> w27
    frame 0, Default {
      # "Not a valid station. Do nothing"
    }
    frame 1 {
      n131 = Bundle By Name(cluster=w600, "Station Test State 1"=w599) -> (w598:T1)
    }
    frame 2 {
      n132 = Bundle By Name(cluster=w603, "Station Test State 2"=w601) -> (w602:T1)
    }
    frame 3 {
      n133 = Bundle By Name(cluster=w606, "Station Test State 3"=w604) -> (w605:T1)
    }
    frame 4 {
      n134 = Bundle By Name(cluster=w609, "Station Test State 4"=w607) -> (w608:T1)
    }
    frame 5 {
      n135 = Bundle By Name(cluster=w612, "Station Test State 5"=w610) -> (w611:T1)
    }
    frame 6 {
      n136 = Bundle By Name(cluster=w615, "Station Test State 6"=w613) -> (w614:T1)
    }
    frame 7 {
      n137 = Bundle By Name(cluster=w618, "Station Test State 7"=w616) -> (w617:T1)
    }
    frame 8 {
      n138 = Bundle By Name(cluster=w621, "Station Test State 8"=w619) -> (w620:T1)
    }
    frame 9 {
      n139 = Bundle By Name(cluster=w624, "Station Test State 9"=w622) -> (w623:T1)
    }
    frame 10 {
      n140 = Bundle By Name(cluster=w627, "Station Test State 10"=w625) -> (w626:T1)
    }
    frame 11 {
      n141 = Bundle By Name(cluster=w630, "Station Test State 11"=w628) -> (w629:T1)
    }
    frame 12 {
      n142 = Bundle By Name(cluster=w633, "Station Test State 12"=w631) -> (w632:T1)
    }
    frame 13 {
      n143 = Bundle By Name(cluster=w636, "Station Test State 13"=w634) -> (w635:T1)
    }
    frame 14 {
      n144 = Bundle By Name(cluster=w639, "Station Test State 14"=w637) -> (w638:T1)
    }
    frame 15 {
      n145 = Bundle By Name(cluster=w642, "Station Test State 15"=w640) -> (w641:T1)
    }
    frame 16 {
      n146 = Bundle By Name(cluster=w645, "Station Test State 16"=w643) -> (w644:T1)
    }
    frame 17 {
      n147 = Bundle By Name(cluster=w648, "Station Test State 17"=w646) -> (w647:T1)
    }
    frame 18 {
      n148 = Bundle By Name(cluster=w651, "Station Test State 18"=w649) -> (w650:T1)
    }
    frame 19 {
      n149 = Bundle By Name(cluster=w654, "Station Test State 19"=w652) -> (w653:T1)
    }
    frame 20 {
      n150 = Bundle By Name(cluster=w657, "Station Test State 20"=w655) -> (w656:T1)
    }
    frame 21 {
      n151 = Bundle By Name(cluster=w660, "Station Test State 21"=w658) -> (w659:T1)
    }
    frame 22 {
      n152 = Bundle By Name(cluster=w663, "Station Test State 22"=w661) -> (w662:T1)
    }
    frame 23 {
      n153 = Bundle By Name(cluster=w666, "Station Test State 23"=w664) -> (w665:T1)
    }
    frame 24 {
      n154 = Bundle By Name(cluster=w669, "Station Test State 24"=w667) -> (w668:T1)
    }
    frame 25 {
      n155 = Bundle By Name(cluster=w672, "Station Test State 25"=w670) -> (w671:T1)
    }
    frame 26 {
      n156 = Bundle By Name(cluster=w675, "Station Test State 26"=w673) -> (w674:T1)
    }
    frame 27 {
      n157 = Bundle By Name(cluster=w678, "Station Test State 27"=w676) -> (w677:T1)
    }
    frame 28 {
      n158 = Bundle By Name(cluster=w681, "Station Test State 28"=w679) -> (w680:T1)
    }
    frame 29 {
      n159 = Bundle By Name(cluster=w684, "Station Test State 29"=w682) -> (w683:T1)
    }
    frame 30 {
      n160 = Bundle By Name(cluster=w687, "Station Test State 30"=w685) -> (w686:T1)
    }
    frame 31 {
      n161 = Bundle By Name(cluster=w690, "Station Test State 31"=w688) -> (w689:T1)
    }
    frame 32 {
      n162 = Bundle By Name(cluster=w693, "Station Test State 32"=w691) -> (w692:T1)
    }
    frame 33 {
      n163 = Bundle By Name(cluster=w696, "Station Test State 33"=w694) -> (w695:T1)
    }
    frame 34 {
      n164 = Bundle By Name(cluster=w699, "Station Test State 34"=w697) -> (w698:T1)
    }
    frame 35 {
      n165 = Bundle By Name(cluster=w702, "Station Test State 35"=w700) -> (w701:T1)
    }
    frame 36 {
      n166 = Bundle By Name(cluster=w705, "Station Test State 36"=w703) -> (w704:T1)
    }
    frame 37 {
      n167 = Bundle By Name(cluster=w708, "Station Test State 37"=w706) -> (w707:T1)
    }
    frame 38 {
      n168 = Bundle By Name(cluster=w711, "Station Test State 38"=w709) -> (w710:T1)
    }
    frame 39 {
      n169 = Bundle By Name(cluster=w714, "Station Test State 39"=w712) -> (w713:T1)
    }
    frame 40 {
      n170 = Bundle By Name(cluster=w717, "Station Test State 40"=w715) -> (w716:T1)
    }
    frame 41 {
      n171 = Bundle By Name(cluster=w720, "Station Test State 41"=w718) -> (w719:T1)
    }
    frame 42 {
      n172 = Bundle By Name(cluster=w723, "Station Test State 42"=w721) -> (w722:T1)
    }
    frame 43 {
      n173 = Bundle By Name(cluster=w726, "Station Test State 43"=w724) -> (w725:T1)
    }
    frame 44 {
      n174 = Bundle By Name(cluster=w729, "Station Test State 44"=w727) -> (w728:T1)
    }
    frame 45 {
      n175 = Bundle By Name(cluster=w732, "Station Test State 45"=w730) -> (w731:T1)
    }
    frame 46 {
      n176 = Bundle By Name(cluster=w735, "Station Test State 46"=w733) -> (w734:T1)
    }
    frame 47 {
      n177 = Bundle By Name(cluster=w738, "Station Test State 47"=w736) -> (w737:T1)
    }
    frame 48 {
      n178 = Bundle By Name(cluster=w741, "Station Test State 48"=w739) -> (w740:T1)
    }
    frame 49 {
      n179 = Bundle By Name(cluster=w744, "Station Test State 49"=w742) -> (w743:T1)
    }
    frame 50 {
      n180 = Bundle By Name(cluster=w747, "Station Test State 50"=w745) -> (w746:T1)
    }
    frame 51 {
      n181 = Bundle By Name(cluster=w750, "Station Test State 51"=w748) -> (w749:T1)
    }
    frame 52 {
      n182 = Bundle By Name(cluster=w753, "Station Test State 52"=w751) -> (w752:T1)
    }
    frame 53 {
      n183 = Bundle By Name(cluster=w756, "Station Test State 53"=w754) -> (w755:T1)
    }
    frame 54 {
      n184 = Bundle By Name(cluster=w759, "Station Test State 54"=w757) -> (w758:T1)
    }
    frame 55 {
      n185 = Bundle By Name(cluster=w762, "Station Test State 55"=w760) -> (w761:T1)
    }
    frame 56 {
      n186 = Bundle By Name(cluster=w765, "Station Test State 56"=w763) -> (w764:T1)
    }
  }
  "Step 2 Output" <- w27
